vi "velocity-unit-subvi-v2.vi"(0 "Axis Select":u8(slide)=1 min=1 max=3 step=1 scale=1.0..3.0, 5 "Input":dbl, 7 "Unit":T1(ring), 11 "error in (no error)":errorcluster) -> (4 "output in counts":dbl, 6 "Unit":T1(ring), 8 "unit":string, 10 "Length and Unit":string, 15 "error out":errorcluster)   [LabVIEW 2009]
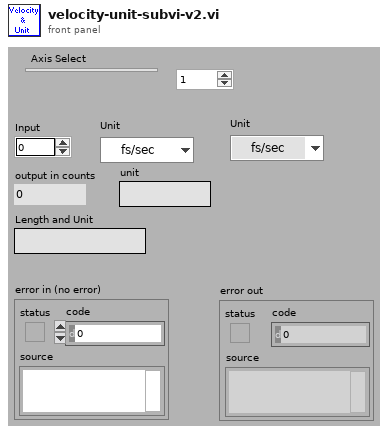
[diagram p1: front panel]
types:
  T1 = enum16{"fs/sec", "ps/sec", "um/sec", "mm/sec", "counts/sec"}
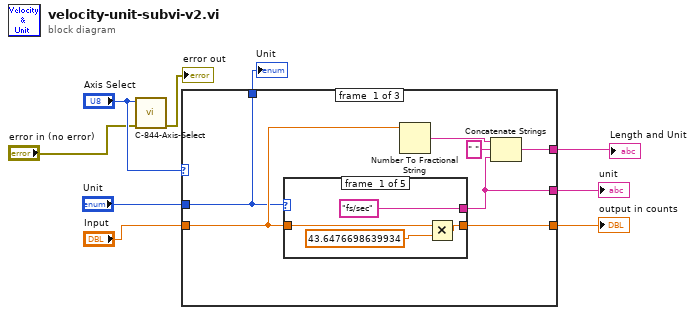
[diagram p0: block diagram]
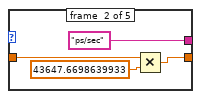
[diagram p2: hidden frame]
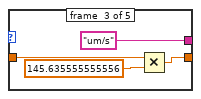
[diagram p3: hidden frame]
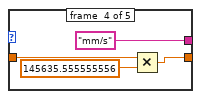
[diagram p4: hidden frame]
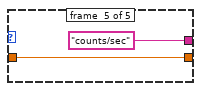
[diagram p5: hidden frame]
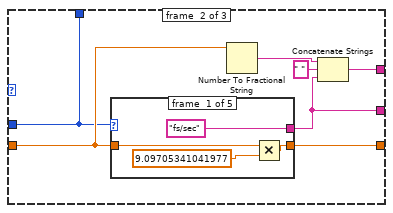
[diagram p6: hidden frame]
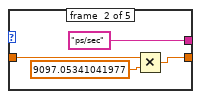
[diagram p7: hidden frame]
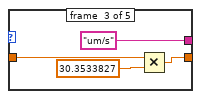
[diagram p8: hidden frame]
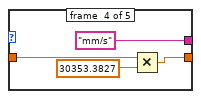
[diagram p9: hidden frame]
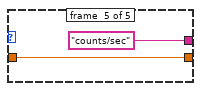
[diagram p10: hidden frame]
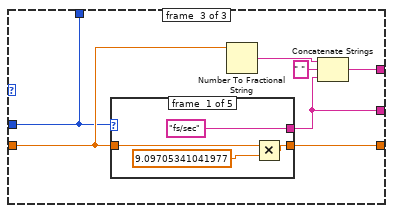
[diagram p11: hidden frame]
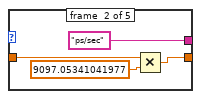
[diagram p12: hidden frame]
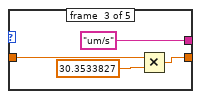
[diagram p13: hidden frame]
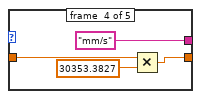
[diagram p14: hidden frame]
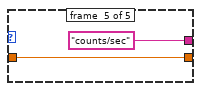
[diagram p15: hidden frame]
diagram:
  n1 = call "C-844-Axis-Select.vi"("error in (no error)"="error in (no error)", "Axis Select"="Axis Select") -> ("error out"=→"error out":errorcluster)  [unwired: 8 in, 1 out]
  n2 = case shown="1, Default" "Axis Select" {
    tunnel: "Unit" -> [w13 w35 w63]
    tunnel: [w10 w41 w62] -> w8
    tunnel: [w12 w38 w60] -> w7
    tunnel: "Input" -> [w14 w37 w64]
    tunnel: [w11 w36 w61] -> w5
    tunnel: [w13 w35 w63] -> w3
    frame #0 {
      n3 = case shown="\"fs/sec\", Default" w13 {
        tunnel: w14 -> [w20 w23 w26 w31 w34]
        tunnel: [w19 w22 w27 w30 w34] -> w10
        tunnel: ["fs/sec" "ps/sec" "um/s" "mm/s" "counts/sec"] -> w11
        frame #0 {
          n4 = Multiply(x=w20, y=43.6476698639934) -> (x*y=w19:dbl)
        }
        frame #1 {
          n5 = Multiply(x=w23, y=43647.6698639933) -> (x*y=w22:dbl)
        }
        frame #2 {
          n6 = Multiply(x=w26, y=145.635555555556) -> (x*y=w27:dbl)
        }
        frame #3 {
          n7 = Multiply(x=w31, y=145635.555555556) -> (x*y=w30:dbl)
        }
        frame #4 {
        }
      }
      n8 = Number To Fractional String(number=w14) -> (F-format string=w16:string)  [unwired: 3 in]
      n9 = Concatenate Strings(w16, " " ("string"), w11) -> (w12:string)
    }
    frame #1 {
      n10 = case shown="\"mm/sec\"" w35 {
        tunnel: w37 -> [w45 w48 w51 w56 w59]
        tunnel: [w44 w47 w52 w55 w59] -> w41
        tunnel: ["fs/sec" "ps/sec" "um/s" "mm/s" "counts/sec"] -> w36
        frame #0 {
          n11 = Multiply(x=w45, y=9.09705341041977) -> (x*y=w44:dbl)
        }
        frame #1 {
          n12 = Multiply(x=w48, y=9097.05341041977) -> (x*y=w47:dbl)
        }
        frame #2 {
          n13 = Multiply(x=w51, y=30.3533827) -> (x*y=w52:dbl)
        }
        frame #3 {
          n14 = Multiply(x=w56, y=30353.3827) -> (x*y=w55:dbl)
        }
        frame #4 {
        }
      }
      n15 = Number To Fractional String(number=w37) -> (F-format string=w40:string)  [unwired: 3 in]
      n16 = Concatenate Strings(w40, " " ("string"), w36) -> (w38:string)
    }
    frame #2 {
      n17 = case shown="\"um/sec\"" w63 {
        tunnel: w64 -> [w70 w73 w76 w81 w84]
        tunnel: [w69 w72 w77 w80 w84] -> w62
        tunnel: ["fs/sec" "ps/sec" "um/s" "mm/s" "counts/sec"] -> w61
        frame #0 {
          n18 = Multiply(x=w70, y=9.09705341041977) -> (x*y=w69:dbl)
        }
        frame #1 {
          n19 = Multiply(x=w73, y=9097.05341041977) -> (x*y=w72:dbl)
        }
        frame #2 {
          n20 = Multiply(x=w76, y=30.3533827) -> (x*y=w77:dbl)
        }
        frame #3 {
          n21 = Multiply(x=w81, y=30353.3827) -> (x*y=w80:dbl)
        }
        frame #4 {
        }
      }
      n22 = Number To Fractional String(number=w64) -> (F-format string=w66:string)  [unwired: 3 in]
      n23 = Concatenate Strings(w66, " " ("string"), w61) -> (w60:string)
    }
  }
  "output in counts" <- w8
  "unit" <- w5
  "Length and Unit" <- w7
  "Unit" <- w3
